vi "cRIO_FPGA_COMMUNICATION Get last Value of Input Data.vi"(8 "Fehler (Eingang, kein Fehler)":errorcluster, 11 "Band Data (Eingang)":bool[][](array[boolean])) -> (0 "Fehler (Ausgang)":errorcluster, 3 "Data (Ausgang)":bool[](array[boolean]))   [LabVIEW 2013, in "cRIO_FPGA_COMMUNICATION.lvlib"]
uses:
  cRIO_FPGA_COMMUNICATION.lvlib
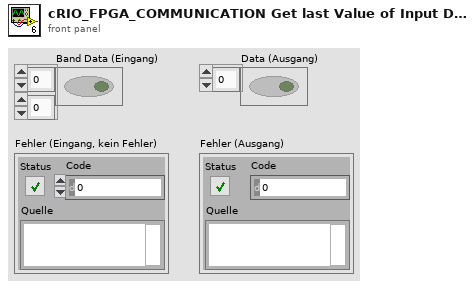
[diagram p1: front panel]
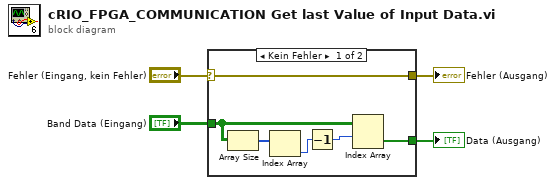
[diagram p0: block diagram]
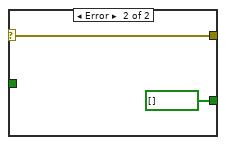
[diagram p2: hidden frame]
diagram:
  n1 = case shown="Kein Fehler" "Fehler (Eingang, kein Fehler)" {
    selector: "Fehler (Eingang, kein Fehler)" -> [w5 w12]
    tunnel: "Band Data (Eingang)" -> [w10 _]
    tunnel: [w6 bool[] [] ("Band Data")] -> w2
    tunnel: [w5 w12] -> w4
    frame No Error {
      n2 = Array Size(array=w10) -> (size(s)=w9:i32[])
      n3 = Index Array(array=w9) -> (element=w8:i32)  [unwired: 1 in]
      n4 = Decrement(x=w8) -> (x-1=w7:i32)
      n5 = Index Array(array=w10, index (row)=w7) -> (element=w6:bool[])  [unwired: 1 in]
    }
    frame Error {
    }
  }
  "Fehler (Ausgang)" <- w4
  "Data (Ausgang)" <- w2
